vi "create raster triangle 2.vi"(10 "object":T2 {"direction" step=0.1}) -> (1 "raster image":bool[][](array[boolean]), 3 "rect":T1)   [LabVIEW 2009]
uses:
  object.ctl
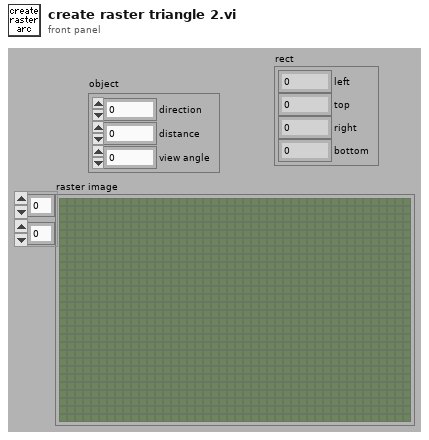
[diagram p1: front panel]
types:
  T1 = cluster{"left":i16, "top":i16, "right":i16, "bottom":i16}
  T2 = typedef "object.ctl" = cluster{"direction":dbl, "distance":u32, "view angle":dbl}
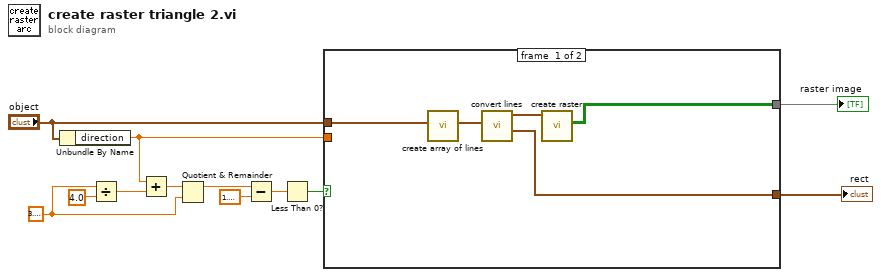
[diagram p0: block diagram]
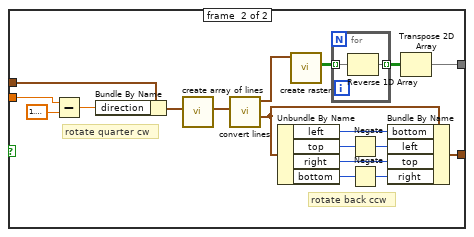
[diagram p2: hidden frame]
diagram:
  w7 = 3.141592653589793
  n1 = Unbundle By Name("object") -> ("direction"=w8:dbl)
  n2 = Divide(x=w7, y=4.0) -> (x/y=w4:dbl)
  n3 = Add(x=w8, y=w4) -> (x+y=w5:dbl)
  n4 = Quotient & Remainder(x=w5, y=w7) -> (x-y*floor(x/y)=w3:dbl)  [unwired: 1 out]
  n5 = Subtract(x=w3, y=1.5707963267948966) -> (x-y=w1:dbl)
  n6 = Less Than 0?(x=w1) -> (x < 0?=w11:bool)
  n7 = case shown="True" w11 {
    tunnel: [w13 w27] -> w12
    tunnel: [w15 w24] -> w10
    tunnel: "object" -> [w14 w33]
    tunnel: w8 -> [_ w31]
    frame #0 {
      n8 = call "create array of lines.vi"("object"=w14) -> ("lines[]"=w16:cluster{"y":i32, "x start":i32, "x end":i32}[])  [unwired: 10 in]
      n9 = call "convert lines.vi"("lines[]"=w16) -> ("rect"=w15:T1, "array (x start, x length)"=w17:cluster{i32, i32}[])  [unwired: 9 in]
      n10 = call "create raster.vi"("Array [x start, x length]"=w17) -> ("raster image"=w13:bool[][])  [unwired: 10 in]
    }
    frame #1 {
      # "rotate back ccw"
      # "rotate quarter cw"
      n11 = Subtract(x=w31, y=1.5707963267948966) -> (x-y=w26:dbl)
      n12 = Bundle By Name(cluster=w33, "direction"=w26) -> (w32:T2)
      n13 = call "create array of lines.vi"("object"=w32) -> ("lines[]"=w34:cluster{"y":i32, "x start":i32, "x end":i32}[])  [unwired: 10 in]
      n14 = call "convert lines.vi"("lines[]"=w34) -> ("rect"=w25:T1, "array (x start, x length)"=w35:cluster{i32, i32}[])  [unwired: 9 in]
      n15 = Unbundle By Name(w25) -> ("left"=w22:i16, "top"=w21:i16, "right"=w23:i16, "bottom"=w19:i16)
      n16 = call "create raster.vi"("Array [x start, x length]"=w35) -> ("raster image"=w29:bool[][])  [unwired: 10 in]
      n17 = for {
        tunnel: w29 -> [w37] mode=indexing
        tunnel: [w36] -> w28 mode=indexing
        n18 = Reverse 1D Array(array=w37) -> (reversed array=w36:bool[])
      }
      n19 = Negate(x=w21) -> (-x=w20:i16)
      n20 = Negate(x=w19) -> (-x=w18:i16)
      n21 = Bundle By Name(cluster=w25, "bottom"=w22, "left"=w20, "top"=w23, "right"=w18) -> (w24:T1)
      n22 = Transpose 2D Array(2D array=w28) -> (transposed array=w27:bool[][])
    }
  }
  "raster image" <- w12
  "rect" <- w10
